vi "GVRefStrom.vi"() -> ()   [LabVIEW 2017]
panel:
  in  "RefStromECD2":i16
  in  "RefStromECD1":i16
  in  "neuerRefstrom":bool
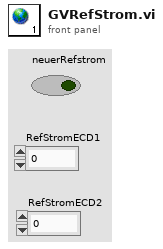
[diagram p1: front panel]
diagram:
